vi "Formula Check.vi"(8 "F(X,t)":string[](array[string])=["t*x1-t+x2", "x1*x2-t"], 9 "X":string[](array[string])=["x1", "x2"], 10 "time":string="t", 11 "X(0)":dbl[](array[numeric]) format="%.2f") -> (0 "system error":bool, 1 "error text":string[](array[string]), 2 "error":i32[](array[numeric]), 3 "error message":string, 5 "result":dbl[][](array[numeric]), 6 "Variables":i32[](array[numeric]), 7 "Table":i32[][][](array[numeric]))   [LabVIEW 2018, in "NI_Gmath.lvlib"]
uses:
  NI_Gmath.lvlib
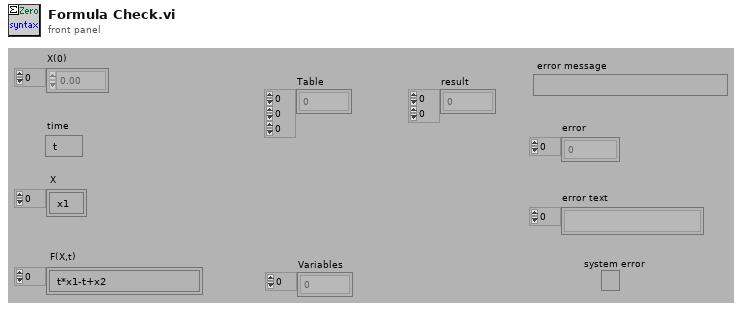
[diagram p1: front panel]
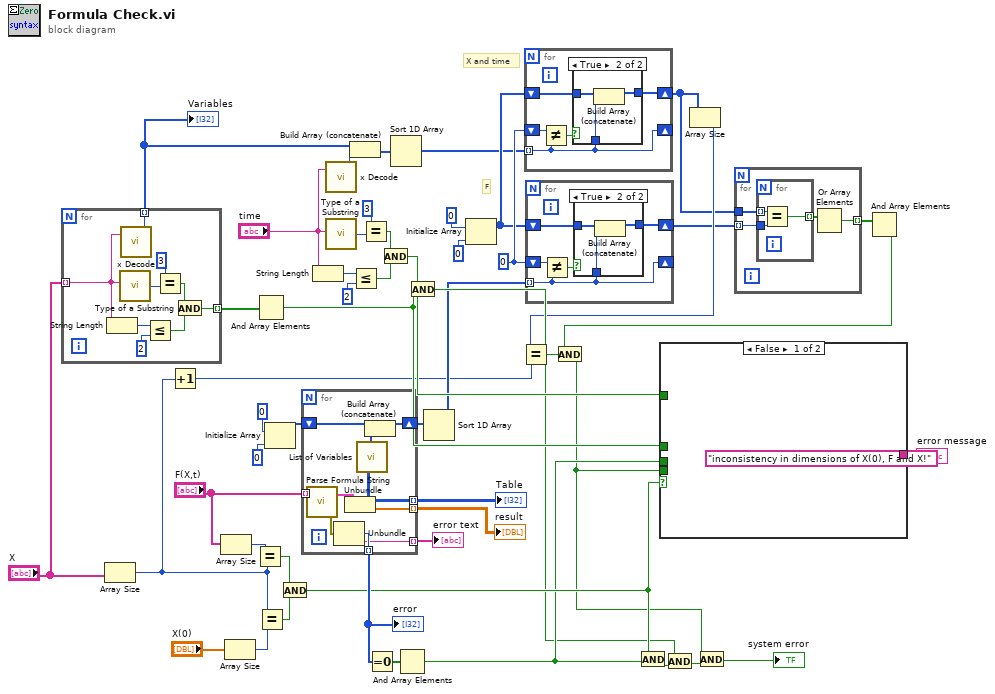
[diagram p0: block diagram]
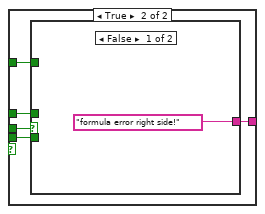
[diagram p4: hidden frame]
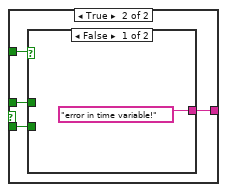
[diagram p5: hidden frame]
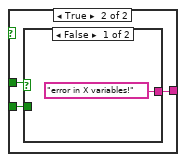
[diagram p6: hidden frame]
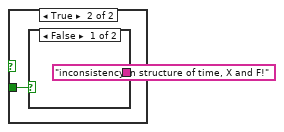
[diagram p7: hidden frame]
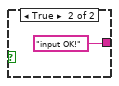
[diagram p8: hidden frame]
diagram:
  w23 = 0
  # "F"
  # "X and time"
  n1 = for {
    tunnel: "X" -> [w53] mode=indexing
    tunnel: [w54] -> w32 mode=indexing
    tunnel: [w52] -> w2 mode=indexing
    n2 = String Length(string=w53) -> (length=w55:i32)
    n3 = call "Type of a Substring.VI"("item"=w53) -> ("type"=w57:i32)
    n4 = call "x Decode.vi"("x string"=w53) -> ("number"=w52:i32)  [unwired: 1 in, 1 out]
    n5 = Less Or Equal?(x=w55, y=2) -> (x <= y?=w59:bool)
    n6 = Equal?(x=3, y=w57) -> (x = y?=w60:bool)
    n7 = And(x=w60, y=w59) -> (x .and. y?=w54:bool)
  }
  "Variables" <- w2
  n8 = Array Size(array="X") -> (size(s)=w17:i32)
  n9 = Increment(x=w17) -> (x+1=w16:i32)
  n10 = Array Size(array="F(X,t)") -> (size(s)=w46:i32)
  n11 = Array Size(array="X(0)") -> (size(s)=w45:i32)
  n12 = Equal?(x=w46, y=w17) -> (x = y?=w43:bool)
  n13 = And Array Elements(Boolean array=w32) -> (logical AND=w30:bool)
  n14 = Equal?(x=w17, y=w45) -> (x = y?=w44:bool)
  n15 = Initialize Array(0, 0) -> (w26:i32[])
  n16 = And(x=w43, y=w44) -> (x .and. y?=w42:bool)
  n17 = for {
    tunnel: [w66] -> w50 mode=indexing
    tunnel: [w61] -> w49 mode=indexing
    tunnel: [w62] -> w48 mode=indexing
    tunnel: "F(X,t)" -> [w70] mode=indexing
    shift-right: [w68] -> w3
    shift-left: w26 -> [w69]
    tunnel: [w65] -> w4 mode=indexing
    n18 = call "Parse Formula String.vi"("formula"=w70) -> ("error out"=w67:errorcluster, "Parsed Formula"=w64:cluster{"Table":i32[][], "Y Values":dbl[]})  [unwired: 1 in]
    n19 = Unbundle(w67) -> ("code"=w66:i32, "source"=w65:string)  [unwired: 1 out]
    n20 = Unbundle(w64) -> ("Table"=w61:i32[][], "Y Values"=w62:dbl[])
    n21 = call "List of Variables.vi"("Table"=w61) -> ("List of variables"=w63:i32[])
    n22 = Build Array (concatenate)(w69, w63) -> (w68:i32[])
  }
  "error" <- w50
  "error text" <- w4
  "result" <- w48
  "Table" <- w49
  n23 = String Length(string="time") -> (length=w39:i32)
  n24 = call "x Decode.vi"("x string"="time") -> ("number"=w21:i32)  [unwired: 1 in, 1 out]
  n25 = call "Type of a Substring.VI"("item"="time") -> ("type"=w37:i32)
  n26 = Build Array (concatenate)(w2, w21) -> (w19:i32[])
  n27 = Less Or Equal?(x=w39, y=2) -> (x <= y?=w35:bool)
  n28 = Equal?(x=3, y=w37) -> (x = y?=w34:bool)
  n29 = Equal To 0?(x=w50) -> (x = 0?=w51:bool[])
  n30 = And(x=w34, y=w35) -> (x .and. y?=w31:bool)
  n31 = Sort 1D Array(array=w19) -> (sorted array=w18:i32[])
  n32 = And Array Elements(Boolean array=w51) -> (logical AND=w40:bool)
  n33 = And(x=w31, y=w30) -> (x .and. y?=w29:bool)
  n34 = Sort 1D Array(array=w3) -> (sorted array=w22:i32[])
  n35 = Initialize Array(0, 0) -> (w20:i32[])
  n36 = for {
    shift-right: [w72] -> w13
    shift-left: w20 -> [w73]
    shift-right: [w71] -> _
    shift-left: w23 -> [w75]
    tunnel: w18 -> [w71] mode=indexing
    n37 = Not Equal?(x=w75, y=w71) -> (x != y?=w74:bool)
    n38 = case shown="True" w74 {
      tunnel: w73 -> [w76 w79]
      tunnel: [w76 w78] -> w72
      tunnel: w71 -> [_ w77]
      frame False {
      }
      frame True {
        n39 = Build Array (concatenate)(w79, w77) -> (w78:i32[])
      }
    }
  }
  n40 = for {
    shift-right: [w81] -> w14
    shift-left: w20 -> [w82]
    shift-right: [w80] -> _
    shift-left: w23 -> [w84]
    tunnel: w22 -> [w80] mode=indexing
    n41 = Not Equal?(x=w84, y=w80) -> (x != y?=w83:bool)
    n42 = case shown="True" w83 {
      tunnel: w82 -> [w85 w88]
      tunnel: [w85 w87] -> w81
      tunnel: w80 -> [_ w86]
      frame False {
      }
      frame True {
        n43 = Build Array (concatenate)(w88, w86) -> (w87:i32[])
      }
    }
  }
  n44 = And(x=w42, y=w40) -> (x .and. y?=w33:bool)
  n45 = And(x=w29, y=w33) -> (x .and. y?=w9:bool)
  n46 = Array Size(array=w13) -> (size(s)=w15:i32)
  n47 = Equal?(x=w15, y=w16) -> (x = y?=w11:bool)
  n48 = for {
    tunnel: w14 -> [w92] mode=indexing
    tunnel: w13 -> [w91]
    tunnel: [w89] -> w12 mode=indexing
    n49 = for {
      tunnel: w92 -> [w95]
      tunnel: w91 -> [w94] mode=indexing
      tunnel: [w93] -> w90 mode=indexing
      n50 = Equal?(x=w94, y=w95) -> (x = y?=w93:bool)
    }
    n51 = Or Array Elements(Boolean array=w90) -> (logical OR=w89:bool)
  }
  n52 = And Array Elements(Boolean array=w12) -> (logical AND=w1:bool)
  n53 = And(x=w1, y=w11) -> (x .and. y?=w10:bool)
  n54 = case shown="False" w42 {
    tunnel: ["inconsistency in dimensions of X(0), F and X!" w101] -> w41
    tunnel: w40 -> [_ w100]
    tunnel: w30 -> [_ w99]
    tunnel: w31 -> [_ w98]
    tunnel: w10 -> [_ w97]
    frame False {
    }
    frame True {
      n55 = case shown="False" w100 {
        tunnel: ["formula error right side!" w106] -> w101
        tunnel: w99 -> [_ w105]
        tunnel: w98 -> [_ w104]
        tunnel: w97 -> [_ w103]
        frame False {
        }
        frame True {
          n56 = case shown="False" w104 {
            tunnel: ["error in time variable!" w110] -> w106
            tunnel: w105 -> [_ w109]
            tunnel: w103 -> [_ w108]
            frame False {
            }
            frame True {
              n57 = case shown="False" w109 {
                tunnel: ["error in X variables!" w113] -> w110
                tunnel: w108 -> [_ w112]
                frame False {
                }
                frame True {
                  n58 = case shown="False" w112 {
                    tunnel: ["inconsistency in structure of time, X and F!" "input OK!"] -> w113
                    frame False {
                    }
                    frame True {
                    }
                  }
                }
              }
            }
          }
        }
      }
    }
  }
  "error message" <- w41
  n59 = And(x=w10, y=w9) -> (x .and. y?=→"system error":bool)
